vi "worksheet set column opt.vi"(5 "options":cluster{"hidden":u8, "level":u8, "collapsed":u8}, 6 "format":u32, 7 "width":dbl, 8 "error in (no error)":errorcluster, 9 "last_col":u16, 10 "first_col":u16, 11 "worksheet":u32) -> (0 "error out":errorcluster, 2 "function return":u32(ring), 3 "options out":cluster{"hidden":u8, "level":u8, "collapsed":u8})   [LabVIEW 2015, in "xlsxwriter.lvlib"]
doc: "lxw_error worksheet_set_column_opt(lxw_worksheet worksheet, lxw_col_t first_col, lxw_col_t last_col, double width, lxw_format format, lxw_row_col_options *options);"
uses:
  xlsxwriter.lvlib
  xlsxwriter.dll
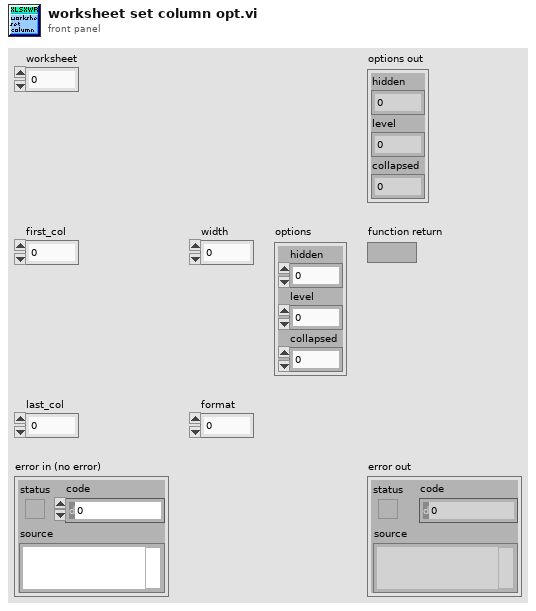
[diagram p1: front panel]
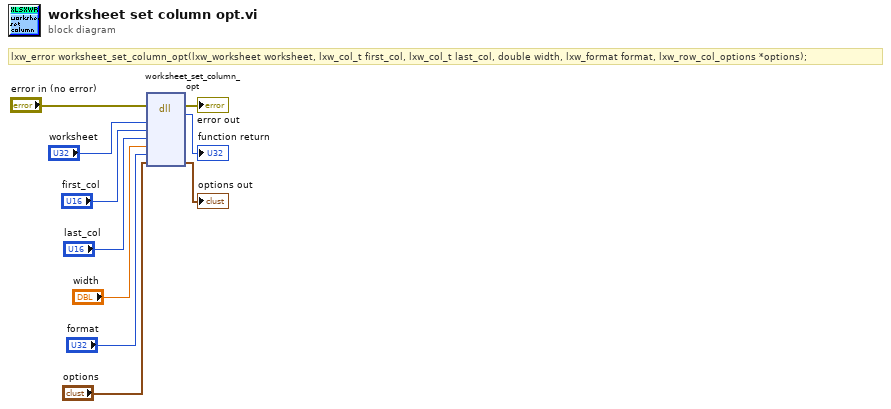
[diagram p0: block diagram]
diagram:
  # "lxw_error worksheet_set_column_opt(lxw_worksheet worksheet, lxw_col_t first_col, lxw_col_t last_col, double width, lxw_format format, lxw_row_col_options *options);"
  n1 = dll-call lib="C:/Users/WDAGUtilityAccount/Desktop/lv_vis_added_cell/xlsxwriter.*" fn="worksheet_set_column_opt"(error in="error in (no error)", "worksheet"="worksheet", "first_col"="first_col", "last_col"="last_col", "width"="width", "format"="format", "options"="options") -> (error out=→"error out":errorcluster, →"function return":u32, "options"=→"options out":cluster{"hidden":u8, "level":u8, "collapsed":u8})  [unwired: 7 in, 1 out]
